vi "Yield (async).vi"(0 "WAMP Client in":refnum<class "WAMP Client.lvclass">, 1 "wamplv.lvlib:Invocation Request.lvclass":refnum<class "Invocation Request ID.lvclass">, 3 "error in (no error)":errorcluster, 4 "Arguments":string, 5 "Options":string, 6 "ArgumentsKw":string) -> (7 "WAMP Client out":refnum<class "WAMP Client.lvclass">, 10 "error out":errorcluster)   [LabVIEW 2020, in "wamplv.lvlib" / "WAMP Client.lvclass"]
uses:
  WAMP Client.lvclass
  Private/Invocation Request ID/Invocation Request ID.lvclass
  Private/TypeDef/YIELD request data.ctl
  Private/TypeDef/Internal Message Type.ctl
  WAMP Client.lvclass/WAMP Client.ctl
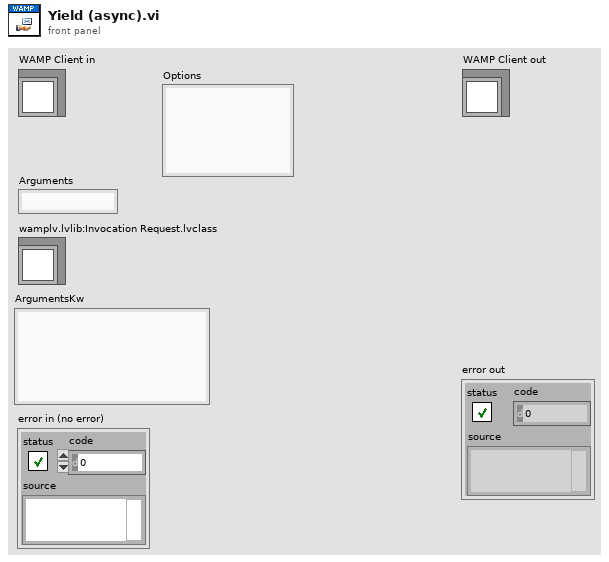
[diagram p1: front panel]
types:
  T1 = typedef "wamplv.lvlib/WAMP Client.lvclass/YIELD request data.ctl" = cluster{"Invocation Request ID":u64, "Arguments":string, "ArgumentsKw":string, "Options":string}
  T2 = typedef "wamplv.lvlib/WAMP Client.lvclass/Internal Message Type.ctl" = enum16{"Subscribe", "Handle Subscribed", "Handle Event", "Unsubscribe", "Handle Unsubscribed", "Publish", "Handled Published", "Goodbye", "Handle Goodbye", "Call", "Handle Result", "Register", "Handle Registered", "Unregister", "Handle Unregistered", "Handle Invocation", "Yield", "Error"}
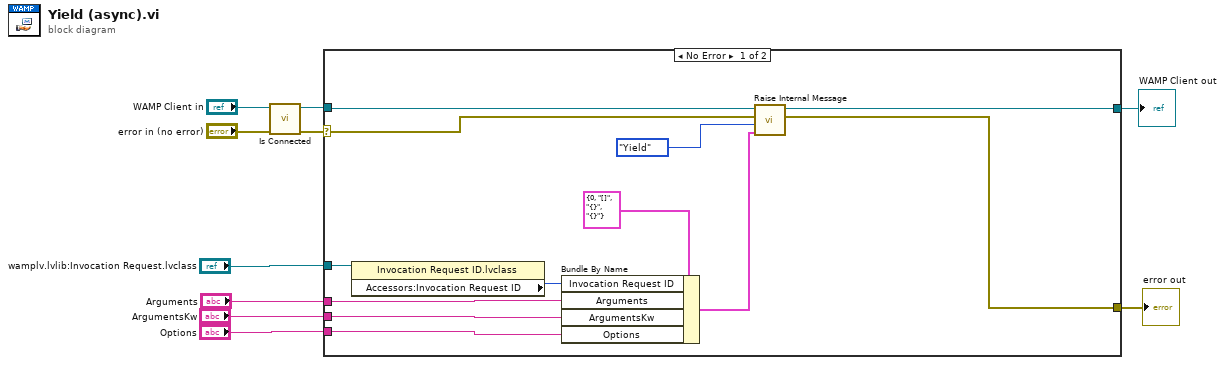
[diagram p0: block diagram]
diagram:
  n1 = call "Is Connected.vi"("error in"="error in (no error)", "WAMP Client in"="WAMP Client in") -> ("error out"=w3:errorcluster, "WAMP Client out"=w4:refnum<class "WAMP Client.lvclass">)  [unwired: 7 in, 1 out]
  n2 = case shown="No Error" w3 {
    selector: w3 -> [w18 w24]
    tunnel: [w19 w24] -> w10
    tunnel: [w21 w23] -> w9
    tunnel: w4 -> [w22 w23]
    tunnel: "ArgumentsKw" -> [w14 _]
    tunnel: "Arguments" -> [w15 _]
    tunnel: "Options" -> [w13 _]
    tunnel: "wamplv.lvlib:Invocation Request.lvclass" -> [w12 _]
    frame No Error {
      n3 = property class="Invocation Request ID.lvclass"(reference=w12) -> ("Accessors:Invocation Request ID"=w11:u64)  [unwired: 1 in, 2 out]
      n4 = Bundle By Name(cluster=T1 {"Invocation Request ID"=0, "Arguments"="[]", "ArgumentsKw"="{}", "Options"="{}"} ("Yield request"), "Invocation Request ID"=w11, "Arguments"=w15, "ArgumentsKw"=w14, "Options"=w13) -> (w16:T1)
      n5 = call "Raise Internal Message.vi"("Variant"=w16, "Internal Message Type"=Internal_Message_Type."Yield", "error in (no error)"=w18, "WAMP Client in"=w22) -> ("error out"=w19:errorcluster, "WAMP Client out"=w21:refnum<class "WAMP Client.lvclass">)  [unwired: 6 in]
    }
    frame Error {
    }
  }
  "error out" <- w10
  "WAMP Client out" <- w9
